vi "Emballage_BDD_Chemins.vi"(8 "error in (no error)":errorcluster, 11 "SetGet":T2=enum."get") -> (0 "error out":errorcluster, 2 "CLT_Chemins_out":T1)   [LabVIEW 2020]
uses:
  Modules/FS/60_FS_Controles/60_FS_SetGet.ctl
panel:
  out "nom":string
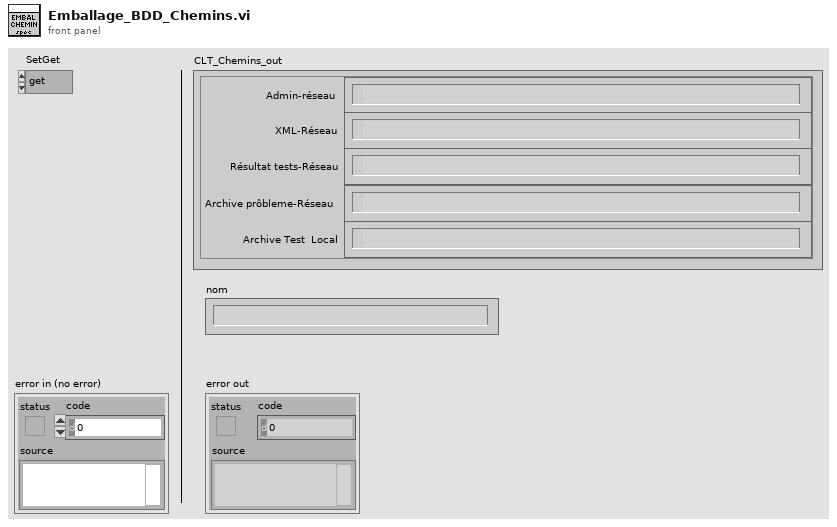
[diagram p1: front panel]
types:
  T1 = cluster{"Admin-réseau":path, "XML-Réseau":path, " Résultat tests-Réseau":path, " Archive prôbleme-Réseau":path, " Archive Test  Local":path}
  T2 = typedef "60_FS_SetGet.ctl" = enum16{"set", "get"}
  T3 = typedef "60_FS_CLT_Chemins.ctl" = cluster{"Racine_local":path, "Racine_reseau":path, "Racine_Support_Application":path, "Fichier_Journalisation":path, "Connexion_BDD_VSX":path, "Connexion_BDD_PLZ":path}
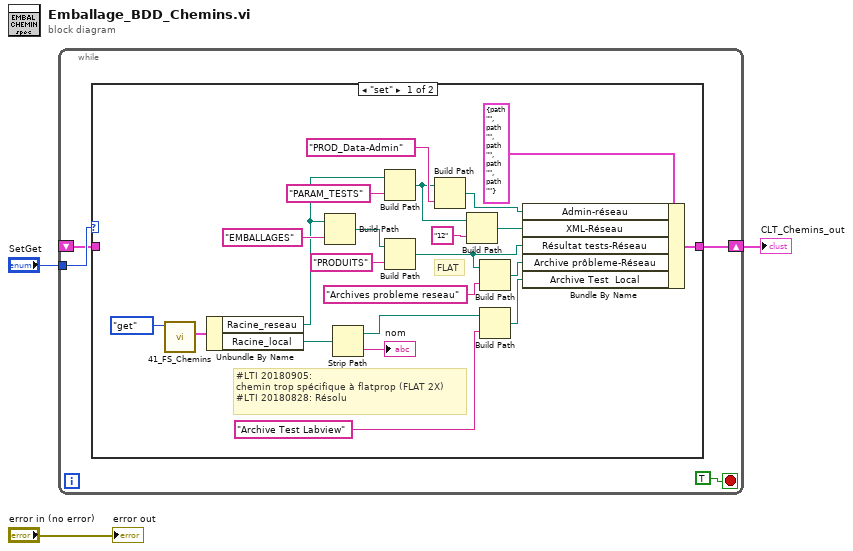
[diagram p0: block diagram]
diagram:
  n1 = while {
    tunnel: "SetGet" -> [w6]
    shift-right: [w5] -> w2
    shift-left: _ -> [w4]
    stop <- TRUE stop-if-true
    n2 = case shown="\"set\"" w6 {
      tunnel: [w27 w30] -> w5
      tunnel: w4 -> [_ w30]
      frame "set" {
        # "FLAT"
        # "#LTI 20180905:\nchemin trop spécifique à flatprop (FLAT 2X)\n#LTI 20180828: Résolu"
        n3 = call "41_FS_Chemins.vi"("SetGet"=60_FS_SetGet."get") -> ("CLT_Chemins_out"=w28:T3)  [unwired: 9 in, 1 out]
        n4 = Unbundle By Name(w28) -> ("Racine_reseau"=w9:path, "Racine_local"=w20:path)
        n5 = Build Path(base path=w9, name or relative path="EMBALLAGES" ("nom ou chemin relatif")) -> (appended path=w10:path)
        n6 = Strip Path(path=w20) -> (stripped path=w19:path, name=→"nom":string)
        n7 = Build Path(base path=w9, name or relative path="PARAM_TESTS" ("nom ou chemin relatif")) -> (appended path=w22:path)
        n8 = Build Path(base path=w10, name or relative path="PRODUITS" ("nom ou chemin relatif")) -> (appended path=w8:path)
        n9 = Build Path(base path=w22, name or relative path="PROD_Data-Admin" ("nom ou chemin relatif")) -> (appended path=w24:path)
        n10 = Build Path(base path=w22, name or relative path="12" ("nom ou chemin relatif")) -> (appended path=w23:path)
        n11 = Build Path(base path=w8, name or relative path="Archives probleme reseau" ("nom ou chemin relatif")) -> (appended path=w13:path)
        n12 = Build Path(base path=w19, name or relative path="Archive Test Labview" ("nom ou chemin relatif")) -> (appended path=w15:path)
        n13 = Bundle By Name(cluster=T1 {"Admin-réseau"=path "", "XML-Réseau"=path "", " Résultat tests-Réseau"=path "", " Archive prôbleme-Réseau"=path "", " Archive Test  Local"=path ""} ("CLT_Chemins_out"), "Admin-réseau"=w24, "XML-Réseau"=w23, "Résultat tests-Réseau"=w8, "Archive prôbleme-Réseau"=w13, "Archive Test  Local"=w15) -> (w27:T1)
      }
      frame "get", Default {
      }
    }
  }
  "CLT_Chemins_out" <- w2
  "error out" <- "error in (no error)"
